vi "Avery Weigth Tronix Get Data.vi"(8 "error in (no error)":errorcluster, 11 "Modbus master in":refnum<class "Modbus Master.lvclass">) -> (0 "error out":errorcluster, 1 "Weight out":T1, 2 "Avery Weigth Tronix Data":string[][](array[string]), 3 "Modbus master out":refnum<class "Modbus Master.lvclass">, 7 "Gross Weight":sgl=29.8)   [LabVIEW 2020]
uses:
  Type Definitions/Avery Weight Tronix Weight.ctl
  <vilib>/NI/Modbus Library/API/Master/Modbus Master.lvclass
panel:
  out "Units":sgl
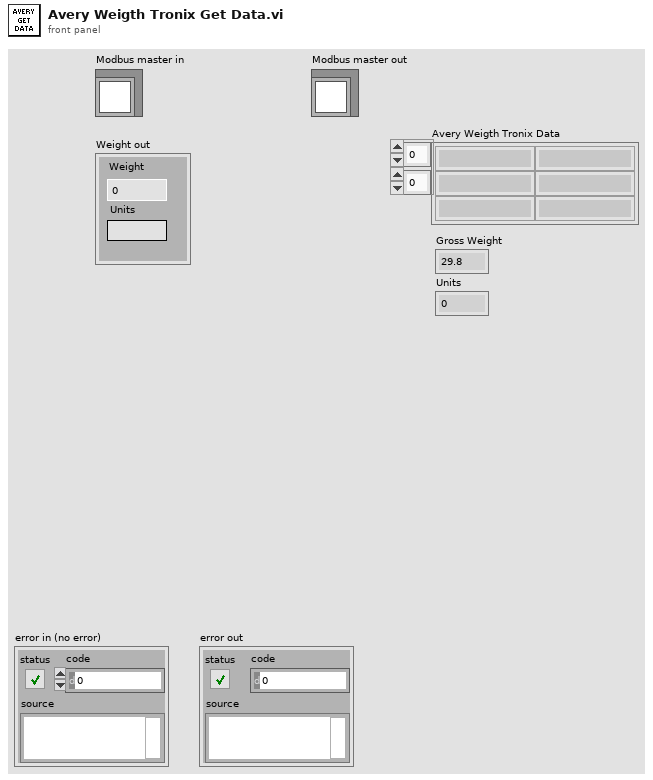
[diagram p1: front panel]
types:
  T1 = typedef "Avery Weight Tronix Weight.ctl" = cluster{"Weight":dbl, "Units":string}
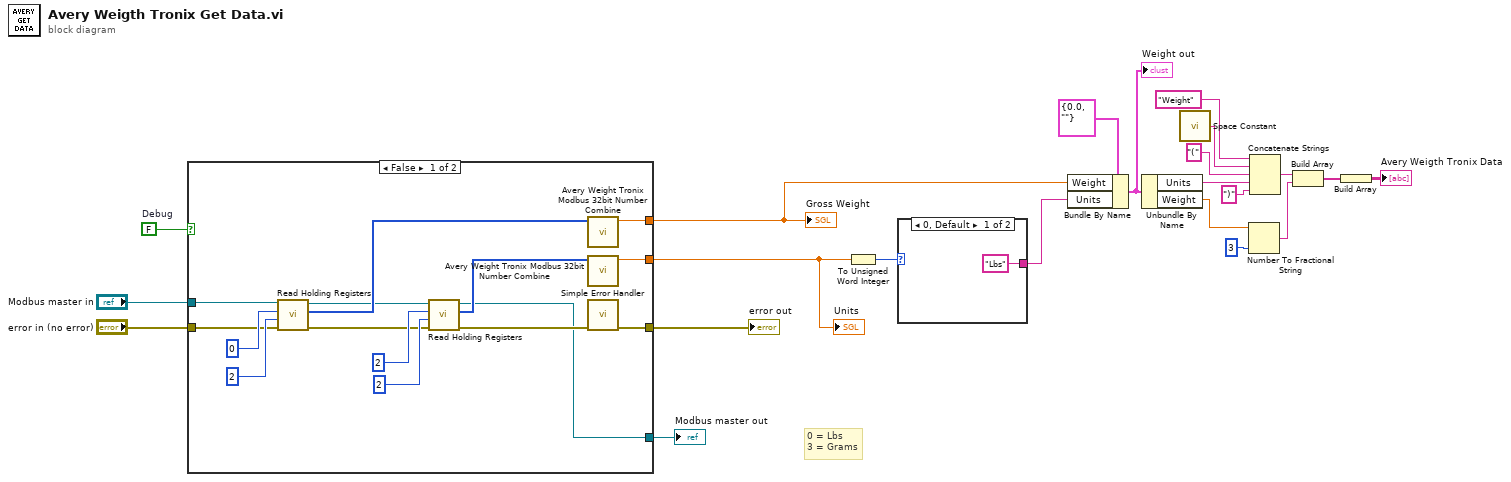
[diagram p0: block diagram]
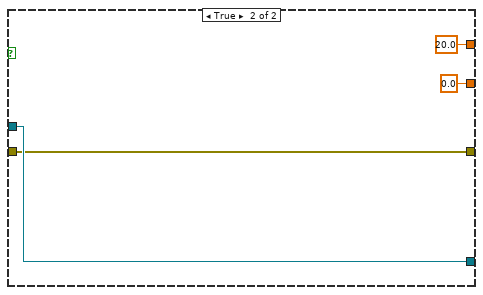
[diagram p2: hidden frame]
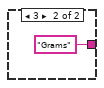
[diagram p3: hidden frame]
diagram:
  w3 = FALSE  # Debug
  # "0 = Lbs\n3 = Grams"
  n1 = case shown="False" w3 {
    tunnel: [w37 w40] -> w22
    tunnel: [w36 sgl 20.0 ("Modbus Float")] -> w11
    tunnel: [w35 sgl 0.0 ("Modbus Float")] -> w7
    tunnel: "error in (no error)" -> [w29 w40]
    tunnel: "Modbus master in" -> [w24 w41]
    tunnel: [w23 w41] -> w4
    frame False {
      n2 = call-dynamic "Read Holding Registers.vi"("error in"=w29, "number of inputs"=u16 2 ("Quantity"), "starting address"=u16 0 ("Starting Address 1"), "Modbus master in"=w24) -> ("error out"=w30:errorcluster, "register values"=w28:u16[], "Modbus master out"=w27:refnum<class "Modbus Master.lvclass">)  [unwired: 5 in]
      n3 = call-dynamic "Read Holding Registers.vi"("error in"=w30, "number of inputs"=u16 2 ("Quantity"), "starting address"=u16 2 ("Starting Address"), "Modbus master in"=w27) -> ("error out"=w26:errorcluster, "register values"=w25:u16[], "Modbus master out"=w23:refnum<class "Modbus Master.lvclass">)  [unwired: 5 in]
      n4 = call "Avery Weight Tronix Modbus 32bit Number Combine.vi"("Holding Registers"=w28) -> ("Modbus Float"=w36:sgl)  [unwired: 9 in, 1 out]
      n5 = call "Avery Weight Tronix Modbus 32bit Number Combine.vi"("Holding Registers"=w25) -> ("Modbus Float"=w35:sgl)  [unwired: 9 in, 1 out]
      n6 = call <vilib>:"Simple Error Handler.vi"("error in (no error)"=w26) -> ("error out"=w37:errorcluster)  [unwired: 1 in, 7 out]
    }
    frame True {
    }
  }
  "Gross Weight" <- w11
  "Units" <- w7
  "error out" <- w22
  "Modbus master out" <- w4
  n7 = To Unsigned Word Integer(number=w7) -> (unsigned 16bit integer=w8:u16)
  n8 = case shown="0, Default" w8 {
    tunnel: ["Lbs" "Grams"] -> w10
    frame 0, Default {
    }
    frame 3 {
    }
  }
  n9 = Bundle By Name(cluster=T1 {"Weight"=0.0, "Units"=""} ("Weight in"), "Weight"=w11, "Units"=w10) -> (w12:T1)
  "Weight out" <- w12
  n10 = Unbundle By Name(w12) -> ("Units"=w18:string, "Weight"=w14:dbl)
  n11 = call <vilib>:"Space Constant.vi"() -> ("String"=w16:string)
  n12 = Number To Fractional String(number=w14, precision (6)=i16 3) -> (F-format string=w21:string)  [unwired: 2 in]
  n13 = Concatenate Strings("Weight" ("string"), w16, "(" ("string"), w18, ")" ("string")) -> (w20:string)
  n14 = Build Array(w20, w21) -> (w2:string[])
  n15 = Build Array(w2) -> (→"Avery Weigth Tronix Data":string[][])
